vi "Read reg.vi"(7 "Read USID":u32=7, 8 "error in (no error)":errorcluster, 10 "Read Address":u32=31, 11 "niDigital in":refnum<class "niDigital.lvclass">) -> (0 "error out":errorcluster, 1 "Read Data Out":u32[][](array[numeric]) format="%.0x", 3 "niDigital out":refnum<class "niDigital.lvclass">)   [LabVIEW 2020, in "niDigital.lvclass"]
uses:
  niDigital.lvclass
  <instrlib>/niDigital/niDigital.llb/niDigital Selected Function.ctl
  <instrlib>/niDigital/niDigital.llb/niDigital Bit Order.ctl
  <instrlib>/niDigital/niDigital.llb/niDigital Data Mapping.ctl
  <instrlib>/niDigital/niDigital.llb/niDigital Create Source Waveform (Serial).vi
  <instrlib>/niDigital/niDigital.llb/niDigital Create Capture Waveform (Serial).vi
  <instrlib>/niDigital/niDigital.llb/niDigital Write Source Waveform (Broadcast U32).vi
  <instrlib>/niDigital/niDigital.llb/niDigital Burst Pattern (Burst Only).vi
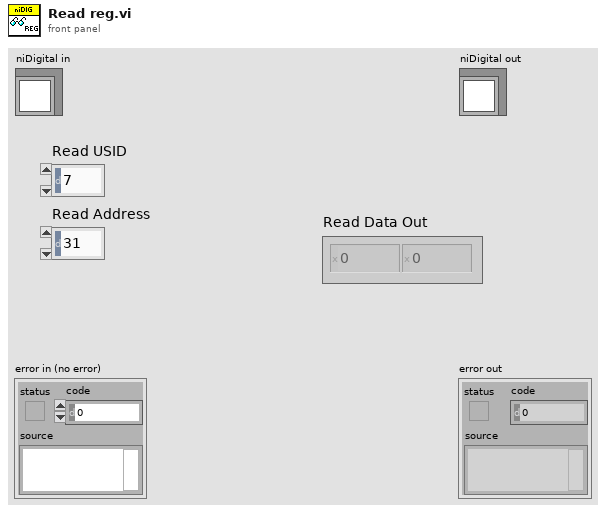
[diagram p1: front panel]
types:
  T1 = typedef "niDigital Data Mapping.ctl" = i32
  T2 = typedef "niDigital Bit Order.ctl" = i32
  T3 = typedef "niDigital Selected Function.ctl" = i32
  T4 = cluster{"Write Reg Pattern":string, "Ext Write Reg Pattern":string, "Cyc Ext Write Reg Pattern":string, "Read Reg Pattern":string}
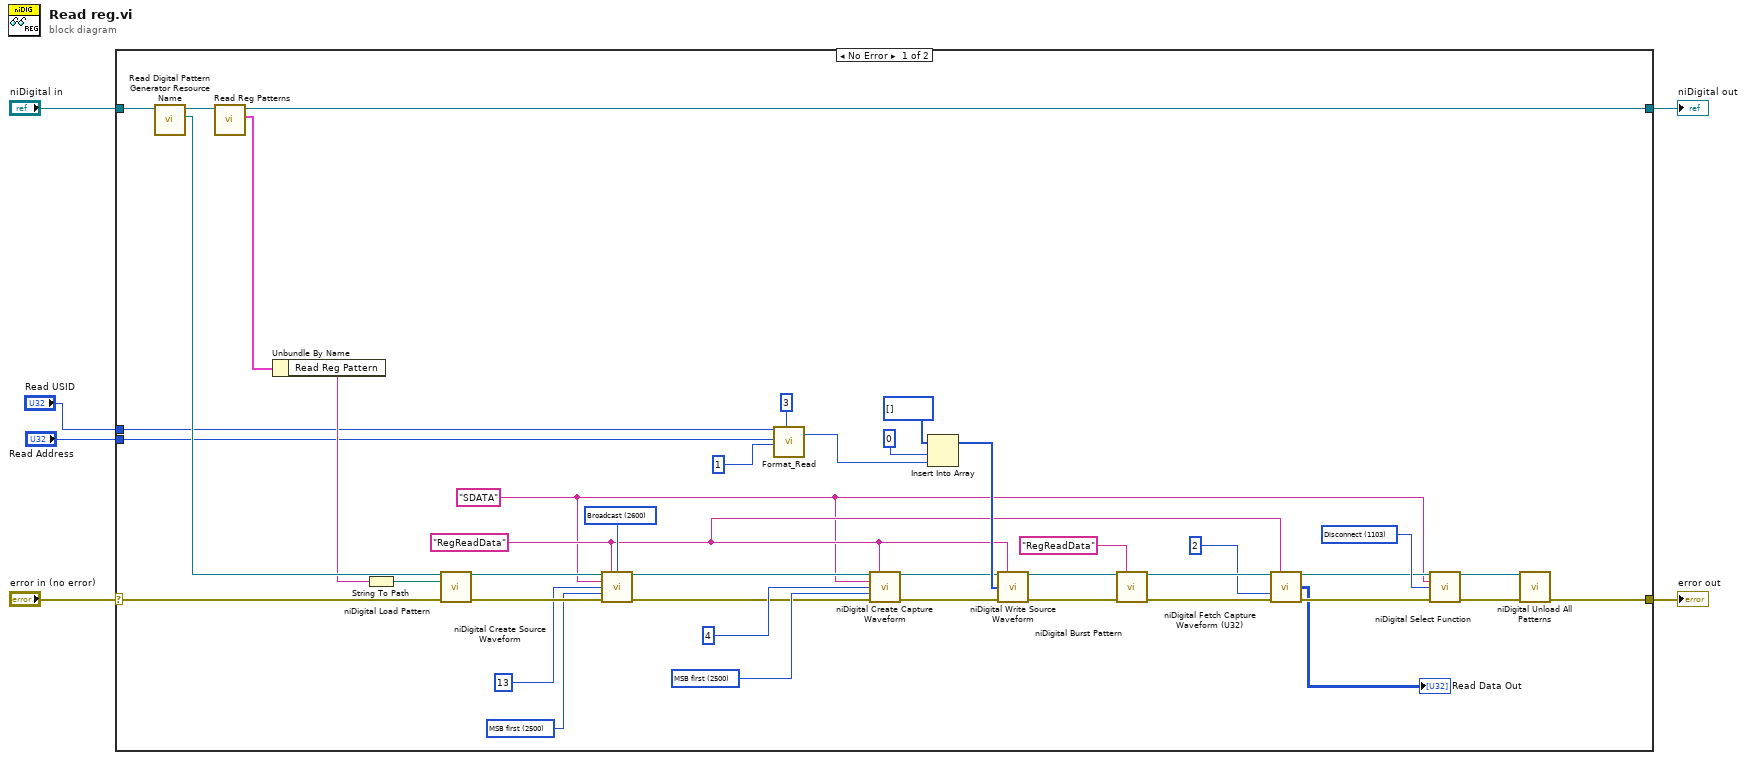
[diagram p0: block diagram]
diagram:
  n1 = case shown="No Error" "error in (no error)" {
    selector: "error in (no error)" -> [w12 w50]
    tunnel: [w13 w50] -> w3
    tunnel: [w46 w49] -> w4
    tunnel: "niDigital in" -> [w48 w49]
    tunnel: "Read Address" -> [w8 _]
    tunnel: "Read USID" -> [w7 _]
    frame No Error {
      w16 = "RegReadData" ("Read waveform name")
      w17 = T1 2600 items=["Broadcast"=2600, "Site Unique"=2601] ("data mapping")
      w22 = T2 2500 items=["MSB first"=2500, "LSB first"=2501] ("bit order")
      w39 = T3 1103 items=["Digital"=1100, "PPMU"=1101, "Off"=1102, "Disconnect"=1103] ("function")
      w15 = "SDATA" ("pin list")
      w43 = T2 2500 items=["MSB first"=2500, "LSB first"=2501] ("bit order")
      n2 = call-dynamic "Read Digital Pattern Generator Resource Name.vi"("niDigital in"=w48) -> ("Digital Pattern Generator Resource Name"=w11:refnum<k15>, "niDigital out"=w47:refnum<class "niDigital.lvclass">)  [unwired: 9 in]
      n3 = call-dynamic "Read Reg Patterns.vi"("niDigital in"=w47) -> ("Reg Patterns"=w10:T4, "niDigital out"=w46:refnum<class "niDigital.lvclass">)  [unwired: 9 in]
      n4 = Unbundle By Name(w10) -> ("Read Reg Pattern"=w9:string)
      n5 = String To Path(string=w9) -> (path=w45:path)
      n6 = call <instrlib>:"niDigital Load Pattern.vi"("instrument handle"=w11, "pattern file"=w45, "error in"=w12) -> ("instrument handle out"=w24:refnum<k15>, "error out"=w25:errorcluster)  [unwired: 11 in]
      n7 = call-poly <instrlib>:"niDigital Create Source Waveform.vi"("instrument handle"=w24, "waveform name"=w16, "data mapping"=w17, "pin list"=w15, "sample width"=u32 13, "bit order"=w22, "error in"=w25) -> ("instrument handle out"=w21:refnum<k15>, "error out"=w20:errorcluster)  [unwired: 7 in]
      n8 = call "Format_Read.vi"("Source Address"=w7, "Address"=w8, "Address Parity"=u32 1, "CMD"=u32 3) -> ("RFFE Read Word"=w29:u32)  [unwired: 14 in, 1 out]
      n9 = call-poly <instrlib>:"niDigital Create Capture Waveform.vi"("instrument handle"=w21, "waveform name"=w16, "pin list"=w15, "sample width"=u32 4, "bit order"=w43, "error in"=w20) -> ("instrument handle out"=w18:refnum<k15>, "error out"=w19:errorcluster)  [unwired: 8 in]
      n10 = Insert Into Array(array=u32[] [], index=0, new element=w29) -> (w28:u32[])
      n11 = call-poly <instrlib>:"niDigital Write Source Waveform.vi"("instrument handle"=w18, "waveform name"=w16, "waveform data"=w28, "error in"=w19) -> ("instrument handle out"=w33:refnum<k15>, "error out"=w32:errorcluster)  [unwired: 10 in]
      n12 = call-poly <instrlib>:"niDigital Burst Pattern.vi"("instrument handle"=w33, "start label"="RegReadData", "error in"=w32) -> ("instrument handle out"=w40:refnum<k15>, "error out"=w41:errorcluster)  [unwired: 11 in]
      n13 = call <instrlib>:"niDigital Fetch Capture Waveform (U32).vi"("instrument handle"=w40, "waveform name"=w16, "samples to read"=2, "error in"=w41) -> ("instrument handle out"=w38:refnum<k15>, "data"=→"Read Data Out":u32[][], "error out"=w37:errorcluster)  [unwired: 9 in]
      n14 = call <instrlib>:"niDigital Select Function.vi"("instrument handle"=w38, "channel list"=w15, "function"=w39, "error in"=w37) -> ("instrument handle out"=w35:refnum<k15>, "error out"=w34:errorcluster)  [unwired: 10 in]
      n15 = call <instrlib>:"niDigital Unload All Patterns.vi"("instrument handle"=w35, "error in"=w34) -> ("error out"=w13:errorcluster)  [unwired: 12 in, 1 out]
    }
    frame Error {
    }
  }
  "error out" <- w3
  "niDigital out" <- w4
